vi "IMAQdx Acquisition Template (Host)withDOG.vi"() -> ()   [LabVIEW 2016]
uses:
  <vilib>/userdefined/High Color/IMAQdx.ctl
  <vilib>/vision/driver/IMAQdx.llb/IMAQdx Acquisition Mode.ctl
  <vilib>/vision/driver/IMAQdx.llb/IMAQdx Buffer Number Mode.ctl
  <vilib>/FPGAPlugInAG/roboRIO/niLvFpga_Open_roboRIO.vi
  <vilib>/rvi/interface/common/dynamic/niFpgaDynamicAddResources.vi
  <vilib>/FPGAPlugInAG/Dynamic/niLvFpga_Download_Dynamic.vi
  <vilib>/FPGAPlugInAG/Dynamic/niLvFpga_Run_Dynamic.vi
  <vilib>/visionFPGA/Basics/Configure Image Transfer to Target/IMAQ FPGA Configure Image Transfer to Target U32.vi
  <vilib>/Utility/error.llb/Error Cluster From Error Code.vi
  <vilib>/rvi/errors/niLvFpgaAdjustHostInterfaceError.vi
  <vilib>/visionFPGA/Basics/Image Transfer to Target/IMAQ FPGA Image Transfer to Target U32.vi
  <vilib>/rvi/interface/common/niFpgaWaitOnOcc.vi
  <vilib>/FPGAPlugInAG/Dynamic/niLvFpga_Close_Dynamic.vi
  <vilib>/rvi/interface/nirviOpenFPGA/nirviOpenFPGA.xnode
  FPGA Bitfiles/ImageProcessingw_FPGATarget2_ImageProcessingw_ZcF2hsHpmf8.lvbitx
  <vilib>/rvi/interface/nirviMethod/nirviMethod.xnode
  <vilib>/rvi/interface/nirviReadWriteControl/nirviReadWriteControl.xnode
  <vilib>/rvi/interface/nirviCloseFPGA/nirviCloseFPGA.xnode
  <vilib>/vision/driver/NI_Vision_Acquisition_Software.lvlib
  <resource>/objmgr/imaqdx.rc
  <vilib>/visionFPGA/NI_VDM_FPGA_Basics.lvlib
  <vilib>/rvi/interface/Simulation/niFpgaSimulationCallBeginRW.vi
  <vilib>/rvi/errors/niLvFpgaMergeErrorWithErrorCode.vi
  <vilib>/FPGAPlugInAG/Dynamic/niLvFpga_ReadFifo_Dynamic.vi
  <vilib>/FPGAPlugInAG/Dynamic/niLvFpga_ConfigureFifo_Dynamic.vi
  <vilib>/FPGAPlugInAG/Dynamic/niLvFpga_StartFifo_Dynamic.vi
  NiFpgaLv.dll
panel:
  out "OriImage Err out":errorcluster
  out "Image":T1(plugin-control)
  out "Count":i32
  out "error out 2":errorcluster
  out "sendPic":bool=TRUE
  in  "Camera":T2
  out "Error Out":errorcluster
  in  "Stop":bool
  # "Overview: Demonstrates how to acquire an image from a camera using the IMAQdx API, transfer the image to a FPGA target for processing, and retrieve the processed image for display or further processing on the host.\nRequirements:\n- LabVIEW FPGA\n- Vision Acquisition Software\n- Vision Development Module\nInstructions:\n1. Select a Camera\n2. Run the VI."
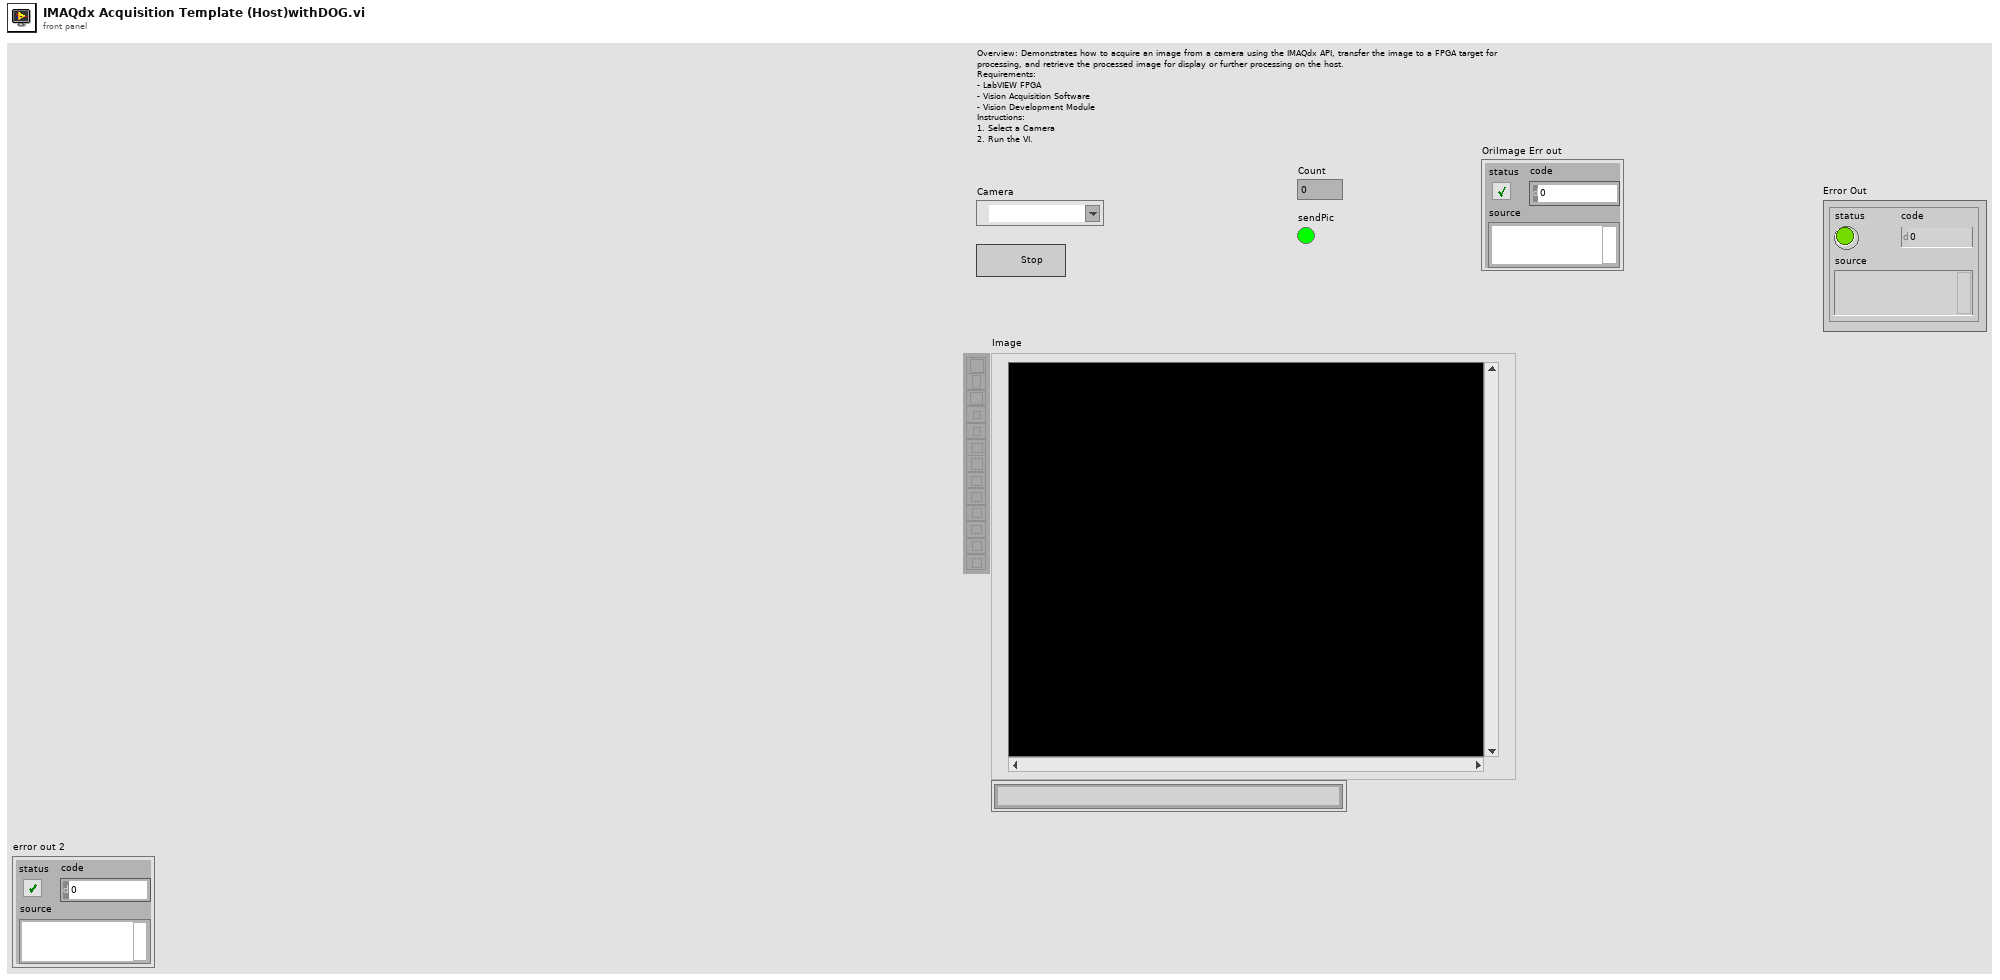
[diagram p1: front panel]
types:
  T1 = typedef "IMAQ Image.ctl" = refnum<image>
  T2 = typedef "IMAQdx.ctl" = refnum<k21>
  T3 = typedef "Image Type" = u32
  T4 = typedef "NI_Vision_Acquisition_Software.lvlib/IMAQdx Acquisition Mode.ctl" = enum32{"One Shot", "Continuous"}
  T5 = typedef "NI_Vision_Acquisition_Software.lvlib/IMAQdx Buffer Number Mode.ctl" = enum32{"Next", "Last", "Buffer Number", "Every", "Last New"}
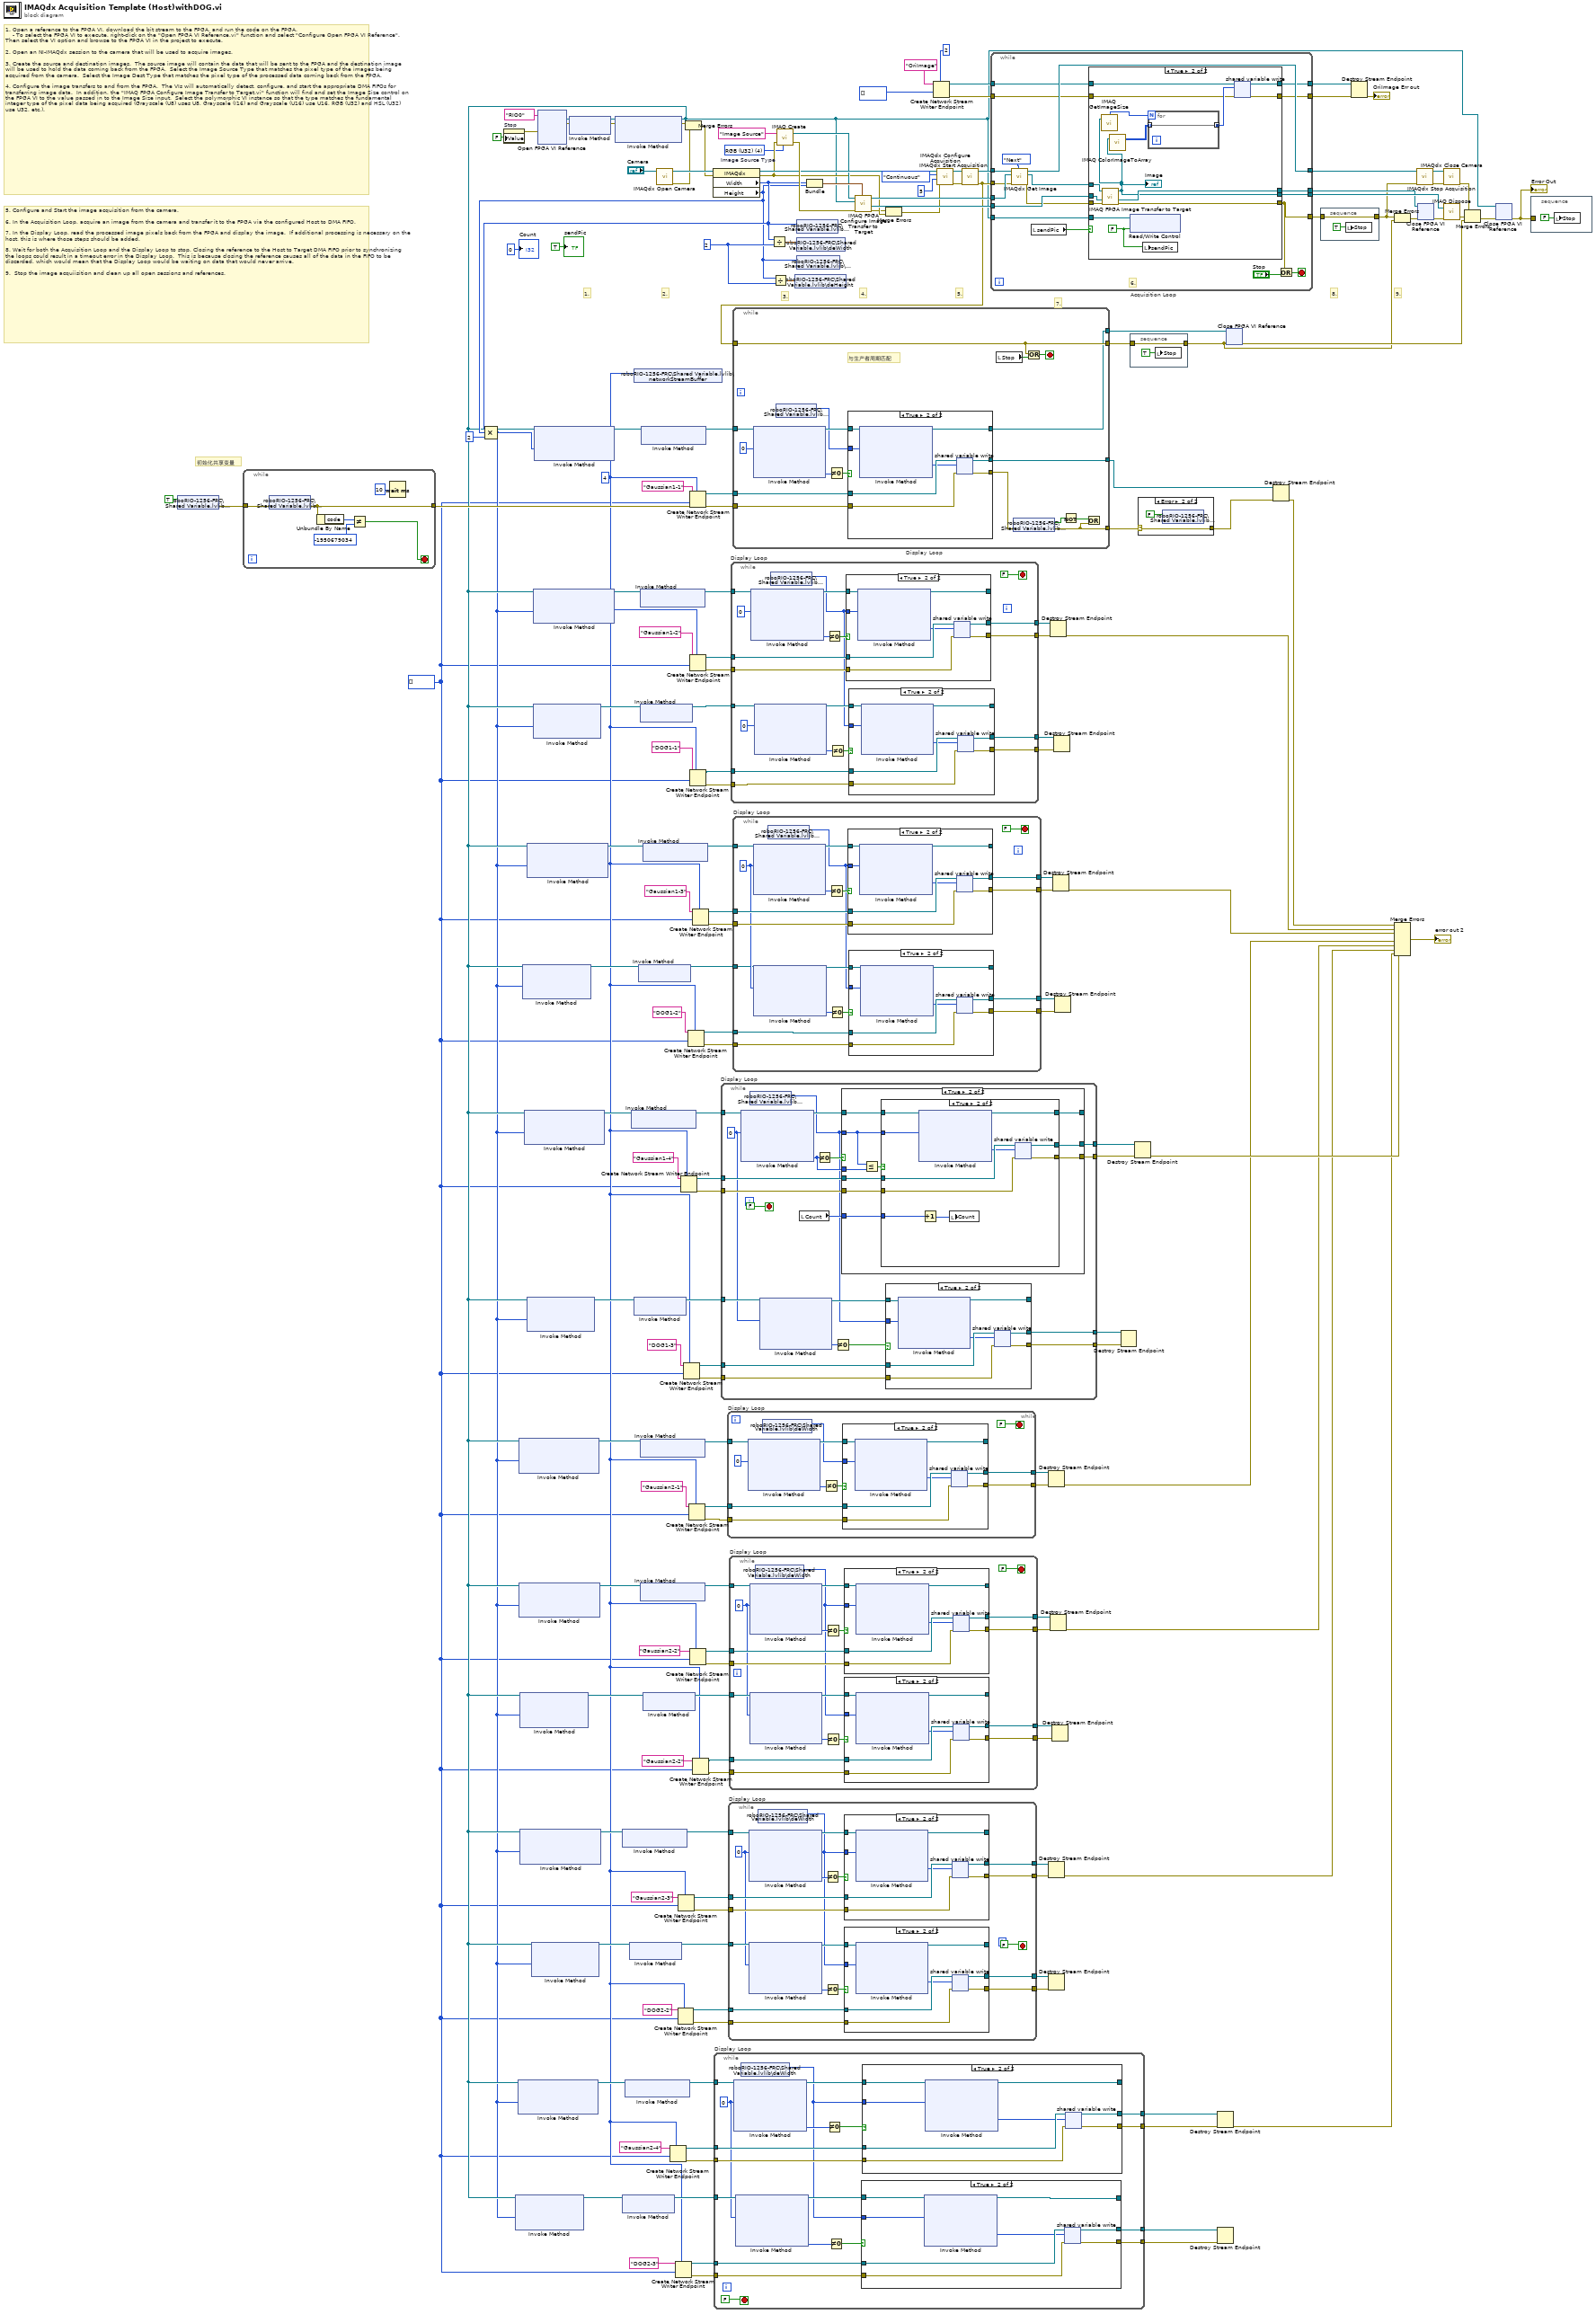
[diagram p0: block diagram]
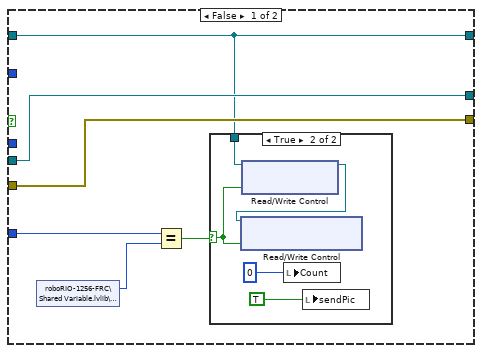
[diagram p8: hidden frame]
diagram:
  w49 = u32 2 ("y")
  w1 = i32[] []
  w2 = 4 ("writer buffer size")
  w140 = T3 4 items=["Grayscale (U8)", "Grayscale (I16)", "Grayscale (SGL)", "Complex (CSG)", "RGB (U32)", "HSL (U32)", "RGB (U64)", "Grayscale (U16)"]  # Image Source Type
  # "初始化共享变量"
  # "5. Configure and Start the image acquisition from the camera.\n\n6. In the Acquisition Loop, acquire an image from the camera and transfer it to the FPGA via the configured Host to DMA FIFO.\n\n7. In the Display Loop, read the processed image pixels back from the FPGA and display the image.  If additional processing is necessary on the host, this is where those steps should be added.\n\n8. Wait for both the Acquisition Loop and the Display Loop to stop. Closing the reference to the Host to Target DMA FIFO prior to synchronizing the loops could result in a timeout error in the Display Loop.  This is because closing the reference causes all of the data in the FIFO to be discarded, which would mean that the Display Loop would be waiting on data that would never arrive.\n\n9.  Stop the image acquiisition and clean up all open sessions and references."
  # "1. Open a reference to the FPGA VI, download the bit stream to the FPGA, and run the code on the FPGA.\n    - To select the FPGA VI to execute, right-click on the \"Open FPGA VI Reference.vi\" function and select \"Configure Open FPGA VI Reference\".  Then select the VI option and browse to the FPGA VI in the project to execute.\n\n2. Open an NI-IMAQdx session to the camera that will be used to acquire images.\n\n3. Create the source and destination images.  The source image will contain the data that will be sent to the FPGA and the destination image will be used to hold the data coming back from the FPGA.  Select the Image Source Type that matches the pixel type of the images being acquired from the camera.  Select the Image Dest Type that matches the pixel type of the processed data coming back from the FPGA.\n\n4. Configure the image transfers to and from the FPGA.  The VIs will automatically detect, configure, and start the appropriate DMA FIFOs for transferring image data.  In addition, the \"IMAQ FPGA Configure Image Transfer to Target.vi\" function will find and set the Image Size control on the FPGA VI to the value passed in to the Image Size input.  Select the polymorphic VI instance so that the type matches the fundamental integer type of the pixel data being acquired (Grayscale (U8) uses U8, Grayscale (I16) and Grayscale (U16) use U16, RGB (U32) and HSL (U32) use U32, etc.)."
  # "9."
  # "8."
  # "7."
  # "6."
  # "5."
  # "4."
  # "3."
  # "2."
  # "1."
  n1 = shared-variable "roboRIO-1256-FRC\\Shared Variable.lvlib\\Active"(TRUE ("Active?")) -> (error out=w126:errorcluster)  [unwired: 1 in]
  n2 = while {
    tunnel: w126 -> [w183]
    tunnel: [w180] -> w125
    stop <- w179 stop-if-true
    n3 = shared-variable "roboRIO-1256-FRC\\Shared Variable.lvlib\\Active"(error in=w183) -> (error out=w180:errorcluster)  [unwired: 1 out]
    n4 = Unbundle By Name(w180) -> ("code"=w182:i32)
    n5 = Not Equal?(x=w182, y=-1950679034) -> (x != y?=w179:bool)
    n6 = Wait (ms)(milliseconds to wait=u32 10) -> ()  [unwired: 1 out]
  }
  n7 = property on="Stop" class="Bool (strict)"("Value"=FALSE ("Stop")) -> (error out=w175:errorcluster)  [unwired: 2 in, 1 out]
  n8 = xnode "Open FPGA VI Reference"("error in"=w175, "resource name"=tag "RIO0") -> ("FPGA VI Reference Out"=w171:refnum<k20>, "error out"=w172:errorcluster)
  n9 = xnode "Invoke Method"("FPGA VI Reference In"=w171, "error in"=w172) -> ("FPGA VI Reference Out"=w174:refnum<k20>, "error out"=w173:errorcluster)
  n10 = xnode "Invoke Method"("FPGA VI Reference In"=w174, "error in"=w173) -> ("FPGA VI Reference Out"=w7:refnum<k20>, "error out"=w160:errorcluster)  [unwired: 1 in]
  n11 = shared-variable "roboRIO-1256-FRC\\Shared Variable.lvlib\\networkStreamBuffer"(w2) -> ()  [unwired: 1 in, 1 out]
  n12 = call <vilib>:"IMAQdx Open Camera.vi"("Session In"="Camera") -> ("error out"=w145:errorcluster, "Session Out"=w146:T2)  [unwired: 9 in]
  n13 = Create Network Stream Writer Endpoint(7:w2, 9:w1, 11:"Gaussian2-4" ("writer name")) -> (0:w87:errorcluster, 3:w88:refnum<k21>)  [unwired: 4 in]
  n14 = Create Network Stream Writer Endpoint(7:w2, 9:w1, 11:"DOG2-3" ("writer name")) -> (0:w3:errorcluster, 3:w4:refnum<k21>)  [unwired: 4 in]
  n15 = Create Network Stream Writer Endpoint(7:w2, 9:w1, 11:"DOG2-2" ("writer name")) -> (0:w38:errorcluster, 3:w39:refnum<k21>)  [unwired: 4 in]
  n16 = Create Network Stream Writer Endpoint(7:w2, 9:w1, 11:"Gaussian2-3" ("writer name")) -> (0:w62:errorcluster, 3:w61:refnum<k21>)  [unwired: 4 in]
  n17 = Create Network Stream Writer Endpoint(7:w2, 9:w1, 11:"Gaussian1-4" ("writer name")) -> (0:w81:errorcluster, 3:w82:refnum<k21>)  [unwired: 4 in]
  n18 = Create Network Stream Writer Endpoint(7:w2, 9:w1, 11:"DOG1-3" ("writer name")) -> (0:w24:errorcluster, 3:w25:refnum<k21>)  [unwired: 4 in]
  n19 = Merge Errors(w160, w145) -> (w144:errorcluster)
  n20 = Create Network Stream Writer Endpoint(7:w2, 9:w1, 11:"DOG1-2" ("writer name")) -> (0:w15:errorcluster, 3:w16:refnum<k21>)  [unwired: 4 in]
  n21 = Create Network Stream Writer Endpoint(7:w2, 9:w1, 11:"Gaussian2-1" ("writer name")) -> (0:w76:errorcluster, 3:w75:refnum<k21>)  [unwired: 4 in]
  n22 = Create Network Stream Writer Endpoint(7:w2, 9:w1, 11:"DOG1-1" ("writer name")) -> (0:w11:errorcluster, 3:w12:refnum<k21>)  [unwired: 4 in]
  n23 = Create Network Stream Writer Endpoint(7:w2, 9:w1, 11:"Gaussian2-2" ("writer name")) -> (0:w69:errorcluster, 3:w70:refnum<k21>)  [unwired: 4 in]
  n24 = Create Network Stream Writer Endpoint(7:w2, 8:w125, 9:w1, 11:"Gaussian1-1" ("writer name")) -> (0:w121:errorcluster, 3:w120:refnum<k21>)  [unwired: 3 in]
  n25 = Create Network Stream Writer Endpoint(7:w2, 9:w1, 11:"Gaussian1-2" ("writer name")) -> (0:w102:errorcluster, 3:w103:refnum<k21>)  [unwired: 4 in]
  n26 = Create Network Stream Writer Endpoint(7:w2, 9:w1, 11:"Gaussian1-3" ("writer name")) -> (0:w97:errorcluster, 3:w96:refnum<k21>)  [unwired: 4 in]
  n27 = Create Network Stream Writer Endpoint(7:w2, 9:w1, 11:"Gaussian2-2" ("writer name")) -> (0:w31:errorcluster, 3:w32:refnum<k21>)  [unwired: 4 in]
  n28 = property class="IMAQdx"(reference=w146, error in=w144) -> (reference out=w153:T2, error out=w141:errorcluster, "Width"=w51:u32, "Height"=w48:u32)
  n29 = Compound Arithmetic op=MULTIPLY(w51, w48, u32 2 ("value")) -> (w6:u32)
  n30 = xnode "Invoke Method"("FPGA VI Reference In"=w7, "Requested Depth"=w6) -> ("FPGA VI Reference Out"=w46:refnum<k20>)  [unwired: 1 in, 2 out]
  n31 = xnode "Invoke Method"("FPGA VI Reference In"=w7, "Requested Depth"=w6) -> ("FPGA VI Reference Out"=w86:refnum<k20>)  [unwired: 1 in, 2 out]
  n32 = xnode "Invoke Method"("FPGA VI Reference In"=w7, "Requested Depth"=w6) -> ("FPGA VI Reference Out"=w58:refnum<k20>)  [unwired: 1 in, 2 out]
  n33 = xnode "Invoke Method"("FPGA VI Reference In"=w7, "Requested Depth"=w6) -> ("FPGA VI Reference Out"=w68:refnum<k20>)  [unwired: 1 in, 2 out]
  n34 = xnode "Invoke Method"("FPGA VI Reference In"=w7, "Requested Depth"=w6) -> ("FPGA VI Reference Out"=w34:refnum<k20>)  [unwired: 1 in, 2 out]
  n35 = xnode "Invoke Method"("FPGA VI Reference In"=w7, "Requested Depth"=w6) -> ("FPGA VI Reference Out"=w63:refnum<k20>)  [unwired: 1 in, 2 out]
  n36 = xnode "Invoke Method"("FPGA VI Reference In"=w7, "Requested Depth"=w6) -> ("FPGA VI Reference Out"=w18:refnum<k20>)  [unwired: 1 in, 2 out]
  n37 = xnode "Invoke Method"("FPGA VI Reference In"=w7, "Requested Depth"=w6) -> ("FPGA VI Reference Out"=w80:refnum<k20>)  [unwired: 1 in, 2 out]
  n38 = xnode "Invoke Method"("FPGA VI Reference In"=w7, "Requested Depth"=w6) -> ("FPGA VI Reference Out"=w27:refnum<k20>)  [unwired: 1 in, 2 out]
  n39 = xnode "Invoke Method"("FPGA VI Reference In"=w7, "Requested Depth"=w6) -> ("FPGA VI Reference Out"=w98:refnum<k20>)  [unwired: 1 in, 2 out]
  n40 = xnode "Invoke Method"("FPGA VI Reference In"=w7, "Requested Depth"=w6) -> ("FPGA VI Reference Out"=w42:refnum<k20>)  [unwired: 1 in, 2 out]
  n41 = xnode "Invoke Method"("FPGA VI Reference In"=w7, "Requested Depth"=w6) -> ("FPGA VI Reference Out"=w14:refnum<k20>)  [unwired: 1 in, 2 out]
  n42 = xnode "Invoke Method"("FPGA VI Reference In"=w7, "Requested Depth"=w6) -> ("FPGA VI Reference Out"=w101:refnum<k20>)  [unwired: 1 in, 2 out]
  n43 = xnode "Invoke Method"("FPGA VI Reference In"=w7, "Requested Depth"=w6) -> ("FPGA VI Reference Out"=w130:refnum<k20>)  [unwired: 1 in, 2 out]
  n44 = xnode "Invoke Method"("FPGA VI Reference In"=w63) -> ("FPGA VI Reference Out"=w64:refnum<k20>)  [unwired: 1 in, 1 out]
  n45 = xnode "Invoke Method"("FPGA VI Reference In"=w46) -> ("FPGA VI Reference Out"=w45:refnum<k20>)  [unwired: 1 in, 1 out]
  n46 = xnode "Invoke Method"("FPGA VI Reference In"=w86) -> ("FPGA VI Reference Out"=w85:refnum<k20>)  [unwired: 1 in, 1 out]
  n47 = xnode "Invoke Method"("FPGA VI Reference In"=w42) -> ("FPGA VI Reference Out"=w40:refnum<k20>)  [unwired: 1 in, 1 out]
  n48 = xnode "Invoke Method"("FPGA VI Reference In"=w80) -> ("FPGA VI Reference Out"=w79:refnum<k20>)  [unwired: 1 in, 1 out]
  n49 = xnode "Invoke Method"("FPGA VI Reference In"=w27) -> ("FPGA VI Reference Out"=w26:refnum<k20>)  [unwired: 1 in, 1 out]
  n50 = xnode "Invoke Method"("FPGA VI Reference In"=w18) -> ("FPGA VI Reference Out"=w17:refnum<k20>)  [unwired: 1 in, 1 out]
  n51 = xnode "Invoke Method"("FPGA VI Reference In"=w14) -> ("FPGA VI Reference Out"=w10:refnum<k20>)  [unwired: 1 in, 1 out]
  n52 = xnode "Invoke Method"("FPGA VI Reference In"=w58) -> ("FPGA VI Reference Out"=w57:refnum<k20>)  [unwired: 1 in, 1 out]
  n53 = xnode "Invoke Method"("FPGA VI Reference In"=w68) -> ("FPGA VI Reference Out"=w67:refnum<k20>)  [unwired: 1 in, 1 out]
  n54 = xnode "Invoke Method"("FPGA VI Reference In"=w101) -> ("FPGA VI Reference Out"=w100:refnum<k20>)  [unwired: 1 in, 1 out]
  n55 = xnode "Invoke Method"("FPGA VI Reference In"=w130) -> ("FPGA VI Reference Out"=w129:refnum<k20>)  [unwired: 1 in, 1 out]
  n56 = xnode "Invoke Method"("FPGA VI Reference In"=w98) -> ("FPGA VI Reference Out"=w99:refnum<k20>)  [unwired: 1 in, 1 out]
  n57 = xnode "Invoke Method"("FPGA VI Reference In"=w34) -> ("FPGA VI Reference Out"=w33:refnum<k20>)  [unwired: 1 in, 1 out]
  n58 = while "Display Loop" {
    tunnel: [w202] -> w91
    tunnel: w87 -> [w201]
    tunnel: w88 -> [w200]
    tunnel: [w196] -> w90
    tunnel: w85 -> [w195]
    tunnel: w45 -> [w192]
    tunnel: w4 -> [w189]
    tunnel: w3 -> [w188]
    tunnel: [w187] -> w44
    tunnel: [w186] -> w43
    stop <- FALSE stop-if-true
    w184 = u32 0 ("Number of Elements")
    n59 = xnode "Invoke Method"("FPGA VI Reference In"=w195, "Number of Elements"=w184) -> ("FPGA VI Reference Out"=w198:refnum<k20>, "Elements Remaining"=w194:u32)  [unwired: 2 in, 2 out]
    n60 = xnode "Invoke Method"("FPGA VI Reference In"=w192, "Number of Elements"=w184) -> ("FPGA VI Reference Out"=w191:refnum<k20>, "Elements Remaining"=w193:u32)  [unwired: 2 in, 2 out]
    n61 = shared-variable "roboRIO-1256-FRC\\Shared Variable.lvlib\\deWidth"() -> (w185:u16)  [unwired: 1 in, 1 out]
    n62 = Not Equal To 0?(x=w194) -> (x != 0?=w199:bool)
    n63 = Not Equal To 0?(x=w193) -> (x != 0?=w190:bool)
    n64 = case shown="True" w190 {
      tunnel: w191 -> [w203 w213]
      tunnel: [w205 w212] -> w187
      tunnel: w188 -> [w204 w211]
      tunnel: w189 -> [w205 w210]
      tunnel: [w204 w209] -> w186
      tunnel: [w203 w208] -> _
      tunnel: w185 -> [_ w207]
      frame False {
      }
      frame True {
        n65 = xnode "Invoke Method"("FPGA VI Reference In"=w213, "Number of Elements"=w207) -> ("FPGA VI Reference Out"=w208:refnum<k20>, "Data"=w206:i16[])  [unwired: 2 in, 2 out]
        n66 = shared-variable-write(w210, w211, w206) -> (w212:refnum<k21>, w209:errorcluster)  [unwired: 1 in, 1 out]
      }
    }
    n67 = case shown="True" w199 {
      tunnel: w198 -> [w214 w224]
      tunnel: [w216 w223] -> w202
      tunnel: w201 -> [w215 w222]
      tunnel: w200 -> [w216 w221]
      tunnel: [w215 w220] -> w196
      tunnel: [w214 w219] -> _
      tunnel: w185 -> [_ w218]
      frame False {
      }
      frame True {
        n68 = xnode "Invoke Method"("FPGA VI Reference In"=w224, "Number of Elements"=w218) -> ("FPGA VI Reference Out"=w219:refnum<k20>, "Data"=w217:u8[])  [unwired: 2 in, 2 out]
        n69 = shared-variable-write(w221, w222, w217) -> (w223:refnum<k21>, w220:errorcluster)  [unwired: 1 in, 1 out]
      }
    }
  }
  n70 = while "Display Loop" {
    tunnel: [w244] -> w84
    tunnel: w81 -> [w243]
    tunnel: w82 -> [w242]
    tunnel: [w238] -> w83
    tunnel: w79 -> [w237]
    tunnel: w26 -> [w233]
    tunnel: w25 -> [w228]
    tunnel: w24 -> [w227]
    tunnel: [w226] -> w23
    tunnel: [w225] -> w22
    stop <- FALSE stop-if-true
    w232 = u32 0 ("Number of Elements")
    n71 = xnode "Invoke Method"("FPGA VI Reference In"=w237, "Number of Elements"=w232) -> ("FPGA VI Reference Out"=w240:refnum<k20>, "Elements Remaining"=w235:u32)  [unwired: 2 in, 2 out]
    n72 = shared-variable "roboRIO-1256-FRC\\Shared Variable.lvlib\\Width"() -> (w229:u16)  [unwired: 1 in, 1 out]
    n73 = xnode "Invoke Method"("FPGA VI Reference In"=w233, "Number of Elements"=w232) -> ("FPGA VI Reference Out"=w231:refnum<k20>, "Elements Remaining"=w234:u32)  [unwired: 2 in, 2 out]
    n74 = local read "Count"() -> (w236:i32)
    n75 = Not Equal To 0?(x=w235) -> (x != 0?=w241:bool)
    n76 = Not Equal To 0?(x=w234) -> (x != 0?=w230:bool)
    n77 = case shown="True" w241 {
      tunnel: w240 -> [w256 w276]
      tunnel: [w261 w275] -> w244
      tunnel: w243 -> [w260 w274]
      tunnel: w242 -> [w261 w273]
      tunnel: [w260 w272] -> w238
      tunnel: [w256 w271] -> _
      tunnel: w229 -> [_ w268]
      tunnel: w236 -> [w258 w270]
      tunnel: w235 -> [_ w267]
      frame False {
        n78 = shared-variable "roboRIO-1256-FRC\\Shared Variable.lvlib\\Height"() -> (w257:u16)  [unwired: 1 in, 1 out]
        n79 = Equal?(x=w258, y=w257) -> (x = y?=w259:bool)
        n80 = case shown="True" w259 {
          selector: w259 -> [_ w263]
          tunnel: w256 -> [_ w266]
          frame False {
          }
          frame True {
            n81 = xnode "Read/Write Control"("FPGA VI Reference In"=w266, "StartOfImage"=w263) -> ("FPGA VI Reference Out"=w265:refnum<k20>)  [unwired: 1 in, 1 out]
            n82 = xnode "Read/Write Control"("FPGA VI Reference In"=w265, "Ready For Output"=w263) -> ()  [unwired: 1 in, 2 out]
            n83 = local write "Count"(0) -> ()
            n84 = local write "sendPic"(TRUE ("start")) -> ()
          }
        }
      }
      frame True {
        n85 = Less Or Equal?(x=w268, y=w267) -> (x <= y?=w269:bool)
        n86 = case shown="True" w269 {
          tunnel: w276 -> [w279 w289]
          tunnel: [w278 w288] -> w275
          tunnel: w274 -> [w277 w287]
          tunnel: w273 -> [w278 w286]
          tunnel: [w277 w285] -> w272
          tunnel: [w279 w283] -> w271
          tunnel: w268 -> [_ w282]
          tunnel: w270 -> [_ w281]
          frame False {
          }
          frame True {
            n87 = xnode "Invoke Method"("FPGA VI Reference In"=w289, "Number of Elements"=w282) -> ("FPGA VI Reference Out"=w283:refnum<k20>, "Data"=w284:u8[])  [unwired: 2 in, 2 out]
            n88 = Increment(x=w281) -> (x+1=w280:i32)
            n89 = local write "Count"(w280) -> ()
            n90 = shared-variable-write(w286, w287, w284) -> (w288:refnum<k21>, w285:errorcluster)  [unwired: 1 in, 1 out]
          }
        }
      }
    }
    n91 = case shown="True" w230 {
      tunnel: w231 -> [w245 w255]
      tunnel: [w247 w254] -> w226
      tunnel: w227 -> [w246 w253]
      tunnel: w228 -> [w247 w252]
      tunnel: [w246 w251] -> w225
      tunnel: [w245 w249] -> _
      tunnel: w229 -> [_ w248]
      frame False {
      }
      frame True {
        n92 = xnode "Invoke Method"("FPGA VI Reference In"=w255, "Number of Elements"=w248) -> ("FPGA VI Reference Out"=w249:refnum<k20>, "Data"=w250:i16[])  [unwired: 2 in, 2 out]
        n93 = shared-variable-write(w252, w253, w250) -> (w254:refnum<k21>, w251:errorcluster)  [unwired: 1 in, 1 out]
      }
    }
  }
  n94 = while "Display Loop" {
    tunnel: [w300] -> w73
    tunnel: w76 -> [w299]
    tunnel: w75 -> [w298]
    tunnel: [w292] -> w74
    tunnel: w57 -> [w291]
    stop <- FALSE stop-if-true
    (unwired) u32 640 ("Number of Elements")
    n95 = xnode "Invoke Method"("FPGA VI Reference In"=w291, "Number of Elements"=u32 0) -> ("FPGA VI Reference Out"=w294:refnum<k20>, "Elements Remaining"=w295:u32)  [unwired: 2 in, 2 out]
    n96 = shared-variable "roboRIO-1256-FRC\\Shared Variable.lvlib\\deWidth"() -> (w290:u16)  [unwired: 1 in, 1 out]
    n97 = Not Equal To 0?(x=w295) -> (x != 0?=w297:bool)
    n98 = case shown="True" w297 {
      tunnel: w294 -> [w301 w311]
      tunnel: [w303 w310] -> w300
      tunnel: w299 -> [w302 w309]
      tunnel: w298 -> [w303 w308]
      tunnel: [w302 w307] -> w292
      tunnel: [w301 w305] -> _
      tunnel: w290 -> [_ w304]
      frame False {
      }
      frame True {
        n99 = xnode "Invoke Method"("FPGA VI Reference In"=w311, "Number of Elements"=w304) -> ("FPGA VI Reference Out"=w305:refnum<k20>, "Data"=w306:u8[])  [unwired: 2 in, 2 out]
        n100 = shared-variable-write(w308, w309, w306) -> (w310:refnum<k21>, w307:errorcluster)  [unwired: 1 in, 1 out]
      }
    }
  }
  n101 = while "Display Loop" {
    tunnel: [w330] -> w59
    tunnel: w62 -> [w329]
    tunnel: w61 -> [w328]
    tunnel: [w323] -> w60
    tunnel: w64 -> [w322]
    tunnel: w40 -> [w317]
    tunnel: w39 -> [w316]
    tunnel: w38 -> [w315]
    tunnel: [w314] -> w37
    tunnel: [w313] -> w36
    stop <- FALSE stop-if-true
    (unwired) u32 640 ("Number of Elements")
    w312 = u32 0 ("Number of Elements")
    (unwired) u32 640 ("Number of Elements")
    n102 = xnode "Invoke Method"("FPGA VI Reference In"=w322, "Number of Elements"=w312) -> ("FPGA VI Reference Out"=w325:refnum<k20>, "Elements Remaining"=w326:u32)  [unwired: 2 in, 2 out]
    n103 = xnode "Invoke Method"("FPGA VI Reference In"=w317, "Number of Elements"=w312) -> ("FPGA VI Reference Out"=w321:refnum<k20>, "Elements Remaining"=w320:u32)  [unwired: 2 in, 2 out]
    n104 = shared-variable "roboRIO-1256-FRC\\Shared Variable.lvlib\\deWidth"() -> (w318:u16)  [unwired: 1 in, 1 out]
    n105 = Not Equal To 0?(x=w326) -> (x != 0?=w327:bool)
    n106 = Not Equal To 0?(x=w320) -> (x != 0?=w319:bool)
    n107 = case shown="True" w327 {
      tunnel: w325 -> [w342 w352]
      tunnel: [w344 w351] -> w330
      tunnel: w329 -> [w343 w350]
      tunnel: w328 -> [w344 w349]
      tunnel: [w343 w348] -> w323
      tunnel: [w342 w346] -> _
      tunnel: w318 -> [_ w345]
      frame False {
      }
      frame True {
        n108 = xnode "Invoke Method"("FPGA VI Reference In"=w352, "Number of Elements"=w345) -> ("FPGA VI Reference Out"=w346:refnum<k20>, "Data"=w347:u8[])  [unwired: 2 in, 2 out]
        n109 = shared-variable-write(w349, w350, w347) -> (w351:refnum<k21>, w348:errorcluster)  [unwired: 1 in, 1 out]
      }
    }
    n110 = case shown="True" w319 {
      tunnel: w321 -> [w331 w341]
      tunnel: [w333 w340] -> w314
      tunnel: w315 -> [w332 w339]
      tunnel: w316 -> [w333 w338]
      tunnel: [w332 w337] -> w313
      tunnel: [w331 w335] -> _
      tunnel: w318 -> [_ w334]
      frame False {
      }
      frame True {
        n111 = xnode "Invoke Method"("FPGA VI Reference In"=w341, "Number of Elements"=w334) -> ("FPGA VI Reference Out"=w335:refnum<k20>, "Data"=w336:i16[])  [unwired: 2 in, 2 out]
        n112 = shared-variable-write(w338, w339, w336) -> (w340:refnum<k21>, w337:errorcluster)  [unwired: 1 in, 1 out]
      }
    }
  }
  n113 = while "Display Loop" {
    tunnel: [w371] -> w72
    tunnel: w69 -> [w370]
    tunnel: w70 -> [w369]
    tunnel: [w364] -> w71
    tunnel: w67 -> [w363]
    tunnel: w33 -> [w358]
    tunnel: w32 -> [w357]
    tunnel: w31 -> [w356]
    tunnel: [w354] -> w30
    tunnel: [w353] -> w29
    stop <- FALSE stop-if-true
    (unwired) u32 640 ("Number of Elements")
    w355 = u32 0 ("Number of Elements")
    (unwired) u32 640 ("Number of Elements")
    n114 = xnode "Invoke Method"("FPGA VI Reference In"=w363, "Number of Elements"=w355) -> ("FPGA VI Reference Out"=w366:refnum<k20>, "Elements Remaining"=w367:u32)  [unwired: 2 in, 2 out]
    n115 = xnode "Invoke Method"("FPGA VI Reference In"=w358, "Number of Elements"=w355) -> ("FPGA VI Reference Out"=w362:refnum<k20>, "Elements Remaining"=w361:u32)  [unwired: 2 in, 2 out]
    n116 = shared-variable "roboRIO-1256-FRC\\Shared Variable.lvlib\\deWidth"() -> (w359:u16)  [unwired: 1 in, 1 out]
    n117 = Not Equal To 0?(x=w367) -> (x != 0?=w368:bool)
    n118 = Not Equal To 0?(x=w361) -> (x != 0?=w360:bool)
    n119 = case shown="True" w368 {
      tunnel: w366 -> [w383 w393]
      tunnel: [w385 w392] -> w371
      tunnel: w370 -> [w384 w391]
      tunnel: w369 -> [w385 w390]
      tunnel: [w384 w389] -> w364
      tunnel: [w383 w387] -> _
      tunnel: w359 -> [_ w386]
      frame False {
      }
      frame True {
        n120 = xnode "Invoke Method"("FPGA VI Reference In"=w393, "Number of Elements"=w386) -> ("FPGA VI Reference Out"=w387:refnum<k20>, "Data"=w388:u8[])  [unwired: 2 in, 2 out]
        n121 = shared-variable-write(w390, w391, w388) -> (w392:refnum<k21>, w389:errorcluster)  [unwired: 1 in, 1 out]
      }
    }
    n122 = case shown="True" w360 {
      tunnel: w362 -> [w372 w382]
      tunnel: [w374 w381] -> w354
      tunnel: w356 -> [w373 w380]
      tunnel: w357 -> [w374 w379]
      tunnel: [w373 w378] -> w353
      tunnel: [w372 w376] -> _
      tunnel: w359 -> [_ w375]
      frame False {
      }
      frame True {
        n123 = xnode "Invoke Method"("FPGA VI Reference In"=w382, "Number of Elements"=w375) -> ("FPGA VI Reference Out"=w376:refnum<k20>, "Data"=w377:u8[])  [unwired: 2 in, 2 out]
        n124 = shared-variable-write(w379, w380, w377) -> (w381:refnum<k21>, w378:errorcluster)  [unwired: 1 in, 1 out]
      }
    }
  }
  n125 = while "Display Loop" {
    tunnel: [w413] -> w110
    tunnel: w102 -> [w412]
    tunnel: w103 -> [w411]
    tunnel: [w405] -> w109
    tunnel: w100 -> [w404]
    tunnel: w12 -> [w398]
    tunnel: w11 -> [w397]
    tunnel: w10 -> [w396]
    tunnel: [w395] -> w9
    tunnel: [w394] -> w8
    stop <- FALSE stop-if-true
    (unwired) u32 640 ("Number of Elements")
    (unwired) u32 640 ("Number of Elements")
    n126 = xnode "Invoke Method"("FPGA VI Reference In"=w404, "Number of Elements"=u32 0) -> ("FPGA VI Reference Out"=w407:refnum<k20>, "Elements Remaining"=w408:u32)  [unwired: 2 in, 2 out]
    n127 = xnode "Invoke Method"("FPGA VI Reference In"=w396, "Number of Elements"=u32 0) -> ("FPGA VI Reference Out"=w403:refnum<k20>, "Elements Remaining"=w402:u32)  [unwired: 2 in, 2 out]
    n128 = shared-variable "roboRIO-1256-FRC\\Shared Variable.lvlib\\Width"() -> (w399:u16)  [unwired: 1 in, 1 out]
    n129 = Not Equal To 0?(x=w408) -> (x != 0?=w410:bool)
    n130 = Not Equal To 0?(x=w402) -> (x != 0?=w400:bool)
    n131 = case shown="True" w410 {
      tunnel: w407 -> [w425 w435]
      tunnel: [w427 w434] -> w413
      tunnel: w412 -> [w426 w433]
      tunnel: w411 -> [w427 w432]
      tunnel: [w426 w431] -> w405
      tunnel: [w425 w429] -> _
      tunnel: w399 -> [_ w428]
      frame False {
      }
      frame True {
        n132 = xnode "Invoke Method"("FPGA VI Reference In"=w435, "Number of Elements"=w428) -> ("FPGA VI Reference Out"=w429:refnum<k20>, "Data"=w430:u8[])  [unwired: 2 in, 2 out]
        n133 = shared-variable-write(w432, w433, w430) -> (w434:refnum<k21>, w431:errorcluster)  [unwired: 1 in, 1 out]
      }
    }
    n134 = case shown="True" w400 {
      tunnel: w403 -> [w414 w424]
      tunnel: [w416 w423] -> w395
      tunnel: w397 -> [w415 w422]
      tunnel: w398 -> [w416 w421]
      tunnel: [w415 w420] -> w394
      tunnel: [w414 w418] -> _
      tunnel: w399 -> [_ w417]
      frame False {
      }
      frame True {
        n135 = xnode "Invoke Method"("FPGA VI Reference In"=w424, "Number of Elements"=w417) -> ("FPGA VI Reference Out"=w418:refnum<k20>, "Data"=w419:i16[])  [unwired: 2 in, 2 out]
        n136 = shared-variable-write(w421, w422, w419) -> (w423:refnum<k21>, w420:errorcluster)  [unwired: 1 in, 1 out]
      }
    }
  }
  n137 = while "Display Loop" {
    tunnel: [w454] -> w93
    tunnel: w97 -> [w453]
    tunnel: w96 -> [w452]
    tunnel: [w447] -> w94
    tunnel: w99 -> [w446]
    tunnel: [w442] -> w21
    tunnel: [w441] -> w20
    tunnel: w17 -> [w438]
    tunnel: w16 -> [w437]
    tunnel: w15 -> [w436]
    stop <- FALSE stop-if-true
    (unwired) u32 640 ("Number of Elements")
    w440 = u32 0 ("Number of Elements")
    (unwired) u32 640 ("Number of Elements")
    n138 = xnode "Invoke Method"("FPGA VI Reference In"=w446, "Number of Elements"=w440) -> ("FPGA VI Reference Out"=w449:refnum<k20>, "Elements Remaining"=w450:u32)  [unwired: 2 in, 2 out]
    n139 = xnode "Invoke Method"("FPGA VI Reference In"=w438, "Number of Elements"=w440) -> ("FPGA VI Reference Out"=w445:refnum<k20>, "Elements Remaining"=w444:u32)  [unwired: 2 in, 2 out]
    n140 = shared-variable "roboRIO-1256-FRC\\Shared Variable.lvlib\\Width"() -> (w439:u16)  [unwired: 1 in, 1 out]
    n141 = Not Equal To 0?(x=w450) -> (x != 0?=w451:bool)
    n142 = Not Equal To 0?(x=w444) -> (x != 0?=w443:bool)
    n143 = case shown="True" w451 {
      tunnel: w449 -> [w466 w476]
      tunnel: [w468 w475] -> w454
      tunnel: w453 -> [w467 w474]
      tunnel: w452 -> [w468 w473]
      tunnel: [w467 w472] -> w447
      tunnel: [w466 w470] -> _
      tunnel: w439 -> [_ w469]
      frame False {
      }
      frame True {
        n144 = xnode "Invoke Method"("FPGA VI Reference In"=w476, "Number of Elements"=w469) -> ("FPGA VI Reference Out"=w470:refnum<k20>, "Data"=w471:u8[])  [unwired: 2 in, 2 out]
        n145 = shared-variable-write(w473, w474, w471) -> (w475:refnum<k21>, w472:errorcluster)  [unwired: 1 in, 1 out]
      }
    }
    n146 = case shown="True" w443 {
      tunnel: w445 -> [w455 w465]
      tunnel: [w457 w464] -> w442
      tunnel: w436 -> [w456 w463]
      tunnel: w437 -> [w457 w462]
      tunnel: [w456 w461] -> w441
      tunnel: [w455 w459] -> _
      tunnel: w439 -> [_ w458]
      frame False {
      }
      frame True {
        n147 = xnode "Invoke Method"("FPGA VI Reference In"=w465, "Number of Elements"=w458) -> ("FPGA VI Reference Out"=w459:refnum<k20>, "Data"=w460:i16[])  [unwired: 2 in, 2 out]
        n148 = shared-variable-write(w462, w463, w460) -> (w464:refnum<k21>, w461:errorcluster)  [unwired: 1 in, 1 out]
      }
    }
  }
  n149 = Divide(x=w51, y=w49) -> (x/y=w50:dbl)
  n150 = Divide(x=w48, y=w49) -> (x/y=w47:dbl)
  n151 = call "IMAQ Create"("Image Name"="Image Source", "Image Type"=w140, "error in (no error)"=w141) -> ("New Image"=w151:T1, "error out"=w159:errorcluster)  [unwired: 2 in]
  n152 = shared-variable "roboRIO-1256-FRC\\Shared Variable.lvlib\\deHeight"(w47) -> ()  [unwired: 1 in, 1 out]
  n153 = shared-variable "roboRIO-1256-FRC\\Shared Variable.lvlib\\Width"(w51) -> ()  [unwired: 1 in, 1 out]
  n154 = shared-variable "roboRIO-1256-FRC\\Shared Variable.lvlib\\deWidth"(w50) -> ()  [unwired: 1 in, 1 out]
  n155 = shared-variable "roboRIO-1256-FRC\\Shared Variable.lvlib\\Height"(w48) -> ()  [unwired: 1 in, 1 out]
  n156 = Bundle("Width"=w51, "Height"=w48) -> (w158:cluster{"Width":u32, "Height":u32})  [unwired: 1 in]
  n157 = call-poly <vilib>:"IMAQ FPGA Configure Image Transfer to Target.vi"("Image Size"=w158, "error in (no error)"=w159, "FPGA VI Reference In"=w7, "Image"=w151) -> ("error out"=w134:errorcluster, "DMA FIFO Reference Out"=w169:refnum<k20>, "Image Out"=w170:T1)  [unwired: 4 in, 1 out]
  n158 = Merge Errors(w134, w141) -> (w133:errorcluster)
  n159 = Create Network Stream Writer Endpoint(7:2 ("writer buffer size"), 9:i32[] [], 11:"OriImage" ("writer name")) -> (0:w114:errorcluster, 3:w115:refnum<k21>)  [unwired: 4 in]
  n160 = call <vilib>:"IMAQdx Configure Acquisition.vi"("error in"=w133, "Number of Buffers"=u32 5, "Continuous?"=IMAQdx_Acquisition_Mode."Continuous", "Session In"=w153) -> ("error out"=w156:errorcluster, "Session Out"=w157:T2)  [unwired: 6 in]
  n161 = call <vilib>:"IMAQdx Start Acquisition.vi"("error in"=w156, "Session In"=w157) -> ("error out"=w132:errorcluster, "Session Out"=w152:T2)  [unwired: 8 in]
  n162 = while "Display Loop" {
    tunnel: w132 -> [w492]
    tunnel: [w480] -> w166
    tunnel: [w492] -> w165
    tunnel: w129 -> [w481]
    tunnel: [w490] -> w123
    tunnel: [w489] -> w122
    tunnel: w121 -> [w488]
    tunnel: w120 -> [w487]
    stop <- w493 stop-if-true
    (unwired) u32 640 ("Number of Elements")
    # "与生产者周期匹配"
    n163 = xnode "Invoke Method"("FPGA VI Reference In"=w481, "Number of Elements"=u32 0) -> ("FPGA VI Reference Out"=w478:refnum<k20>, "Elements Remaining"=w479:u32)  [unwired: 2 in, 2 out]
    n164 = shared-variable "roboRIO-1256-FRC\\Shared Variable.lvlib\\Width"() -> (w477:u16)  [unwired: 1 in, 1 out]
    n165 = Not Equal To 0?(x=w479) -> (x != 0?=w483:bool)
    n166 = case shown="True" w483 {
      tunnel: w478 -> [w494 w504]
      tunnel: [w496 w503] -> w489
      tunnel: w488 -> [w495 w502]
      tunnel: w487 -> [w496 w501]
      tunnel: [w495 w500] -> w486
      tunnel: [w494 w498] -> w480
      tunnel: w477 -> [_ w497]
      frame False {
      }
      frame True {
        n167 = xnode "Invoke Method"("FPGA VI Reference In"=w504, "Number of Elements"=w497) -> ("FPGA VI Reference Out"=w498:refnum<k20>, "Data"=w499:u8[])  [unwired: 2 in, 2 out]
        n168 = shared-variable-write(w501, w502, w499) -> (w503:refnum<k21>, w500:errorcluster)  [unwired: 1 in, 1 out]
      }
    }
    n169 = local read "Stop"() -> (w491:bool)
    n170 = shared-variable "roboRIO-1256-FRC\\Shared Variable.lvlib\\Active"(error in=w486) -> (w484:bool, error out=w490:errorcluster)
    n171 = Or(x=w492, y=w491) -> (x .or. y?=w493:bool)
    n172 = Not(x=w484) -> (.not. x?=w485:bool)
    n173 = Or(x=w485, y=w490) -> ()  [unwired: 1 out]
  }
  n174 = while "Acquisition Loop" {
    tunnel: [w514] -> w138
    tunnel: w170 -> [w519]
    tunnel: w169 -> [w516]
    tunnel: [w515] -> w139
    tunnel: [w512] -> w168
    tunnel: w152 -> [w520]
    tunnel: [w518] -> w148
    tunnel: w132 -> [w517]
    tunnel: w7 -> [w510]
    tunnel: w115 -> [w508]
    tunnel: w114 -> [w507]
    tunnel: [w506] -> w113
    tunnel: [w505] -> w112
    stop <- w522 stop-if-true
    n175 = call <vilib>:"IMAQdx Get Image.vi"("Buffer Number Mode (Next)"=IMAQdx_Buffer_Number_Mode."Next", "error in"=w517, "Image In"=w519, "Session In"=w520) -> ("error out"=w511:errorcluster, "Image Out"=w513:T1, "Session Out"=w518:T2)  [unwired: 4 in, 1 out]
    n176 = local read "sendPic"() -> (w509:bool)
    n177 = case shown="True" w509 {
      tunnel: w516 -> [w528 w543]
      tunnel: [w528 w539] -> w515
      tunnel: [w527 w540] -> w514
      tunnel: w513 -> [w526 w542]
      tunnel: [w526 w534] -> w512
      tunnel: w511 -> [w527 w541]
      tunnel: w510 -> [_ w537]
      tunnel: w508 -> [w525 w532]
      tunnel: w507 -> [w524 w531]
      tunnel: [w525 w530] -> w506
      tunnel: [w524 w529] -> w505
      frame False {
      }
      frame True {
        w538 = FALSE ("EndOfImage")
        n178 = call-poly <vilib>:"IMAQ FPGA Image Transfer to Target.vi"("error in (no error)"=w541, "DMA FIFO Reference In"=w543, "Image"=w542) -> ("error out"=w540:errorcluster, "DMA FIFO Reference Out"=w539:refnum<k20>, "Image Out"=w534:T1)  [unwired: 6 in]
        "Image" <- w534
        n179 = call "IMAQ GetImageSize"("Image"=w534) -> ("X Resolution"=w536:i32)  [unwired: 3 in, 2 out]
        n180 = call "IMAQ ColorImageToArray"("Image"=w534) -> ("Image Pixels (U32)"=w535:u32[][])  [unwired: 3 in, 2 out]
        n181 = xnode "Read/Write Control"("FPGA VI Reference In"=w537, "StartOfImage"=w538) -> ()  [unwired: 1 in, 2 out]
        n182 = local write "sendPic"(w538) -> ()
        n183 = for {
          N: w536 -> [_]
          tunnel: w535 -> [w544] mode=indexing
          tunnel: [w544] -> w533 mode=concatenating
        }
        n184 = shared-variable-write(w532, w531, w533) -> (w530:refnum<k21>, w529:errorcluster)  [unwired: 1 in, 1 out]
      }
    }
    n185 = Or(x=w514, y="Stop") -> (x .or. y?=w522:bool)
  }
  n186 = Destroy Stream Endpoint(8:w74, 11:w73) -> (0:w55:errorcluster)
  n187 = Destroy Stream Endpoint(8:w60, 11:w59) -> (0:w53:errorcluster)
  n188 = Destroy Stream Endpoint(8:w36, 11:w37) -> ()  [unwired: 1 out]
  n189 = Destroy Stream Endpoint(8:w71, 11:w72) -> (0:w54:errorcluster)
  n190 = Destroy Stream Endpoint(8:w109, 11:w110) -> (0:w105:errorcluster)
  n191 = Destroy Stream Endpoint(8:w29, 11:w30) -> ()  [unwired: 1 out]
  n192 = Destroy Stream Endpoint(8:w94, 11:w93) -> (0:w92:errorcluster)
  n193 = Destroy Stream Endpoint(8:w8, 11:w9) -> ()  [unwired: 1 out]
  n194 = Destroy Stream Endpoint(8:w20, 11:w21) -> ()  [unwired: 1 out]
  n195 = Destroy Stream Endpoint(8:w22, 11:w23) -> ()  [unwired: 1 out]
  n196 = stacked-sequence {
    tunnel: w165 -> [w545]
    tunnel: [w545] -> w137
    frame #0 {
      n197 = local write "Stop"(TRUE ("Stop")) -> ()
    }
  }
  n198 = Destroy Stream Endpoint(8:w83, 11:w84) -> (0:w56:errorcluster)
  n199 = case shown="Error" w123 {
    selector: w123 -> [w547 w548]
    tunnel: [w547 w548] -> w108
    frame No Error {
    }
    frame Error {
      n200 = shared-variable "roboRIO-1256-FRC\\Shared Variable.lvlib\\Active"(FALSE ("Active?")) -> ()  [unwired: 1 in, 1 out]
    }
  }
  n201 = Destroy Stream Endpoint(8:w90, 11:w91) -> (0:w52:errorcluster)
  n202 = Destroy Stream Endpoint(8:w43, 11:w44) -> ()  [unwired: 1 out]
  n203 = xnode "Close FPGA VI Reference"("FPGA VI Reference In"=w166, "error in"=w137) -> ("error out"=w164:errorcluster)
  n204 = Destroy Stream Endpoint(8:w108, 11:w122) -> (0:w106:errorcluster)
  n205 = stacked-sequence {
    tunnel: w138 -> [w550]
    tunnel: [w550] -> w135
    frame #0 {
      n206 = local write "Stop"(TRUE ("Stop")) -> ()
    }
  }
  n207 = Destroy Stream Endpoint(8:w112, 11:w113) -> (0:→"OriImage Err out":errorcluster)
  n208 = Merge Errors(w135, w137) -> (w136:errorcluster)
  n209 = Merge Errors(w106, w105, w92, w56, w55, w54, w53, w52) -> (→"error out 2":errorcluster)
  n210 = call <vilib>:"IMAQdx Stop Acquisition.vi"("error in"=w135, "Session In"=w148) -> ("error out"=w149:errorcluster, "Session Out"=w150:T2)  [unwired: 8 in]
  n211 = xnode "Close FPGA VI Reference"("FPGA VI Reference In"=w139, "error in"=w136) -> ("error out"=w167:errorcluster)
  n212 = call <vilib>:"IMAQdx Close Camera.vi"("error in"=w149, "Session In"=w150) -> ("error out"=w147:errorcluster)  [unwired: 9 in]
  n213 = call "IMAQ Dispose"("Image"=w168, "error in (no error)"=w167) -> ("error out"=w163:errorcluster)  [unwired: 4 in]
  n214 = Merge Errors(w147, w163, w164) -> (w143:errorcluster)
  n215 = xnode "Close FPGA VI Reference"("FPGA VI Reference In"=w7, "error in"=w143) -> ("error out"=w142:errorcluster)
  "Error Out" <- w142
  n216 = stacked-sequence {
    tunnel: w142 -> [_]
    frame #0 {
      n217 = local write "Stop"(FALSE ("Stop")) -> ()
    }
  }
  "sendPic" <- TRUE
  "Count" <- 0
